vi "Create Queues.vi"(8 "error in (no error)":errorcluster) -> (0 "error out":errorcluster, 3 "Message Queues Out":T1)   [LabVIEW 2018]
uses:
  Pfizer Timed Seq/Software/support/Message Queue/Message Cluster.ctl
  Pfizer Timed Seq/Software/support/Message Queue/Enqueue Message (Single).vi
  Pfizer Timed Seq/Software/support/Message Queue/Message Queue.lvlib
panel:
  in  "Message Queues In":T1
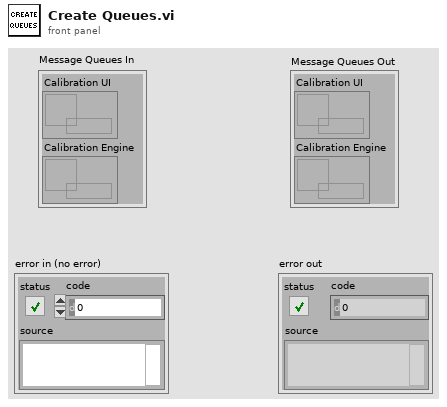
[diagram p1: front panel]
types:
  T1 = cluster{"Calibration UI":refnum<queue>, "Calibration Engine":refnum<queue>}
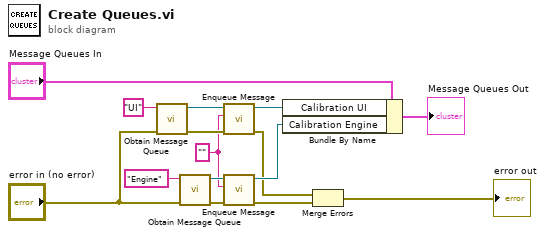
[diagram p0: block diagram]
diagram:
  w1 = "" ("Message")
  n1 = call "Obtain Message Queue.vi"("error in (no error)"="error in (no error)", "name (unnamed)"="UI") -> ("error out"=w12:errorcluster, "Message Queue"=w13:refnum<queue>)  [unwired: 8 in]
  n2 = call "Obtain Message Queue.vi"("error in (no error)"="error in (no error)", "name (unnamed)"="Engine") -> ("error out"=w14:errorcluster, "Message Queue"=w15:refnum<queue>)  [unwired: 8 in]
  n3 = call-poly "Enqueue Message.vi"("error in (no error)"=w12, "Message"=w1, "Message Queue"=w13) -> ("error out"=w4:errorcluster, "dup Message Queue"=w10:refnum<queue>)  [unwired: 7 in]
  n4 = call-poly "Enqueue Message.vi"("error in (no error)"=w14, "Message"=w1, "Message Queue"=w15) -> ("error out"=w3:errorcluster, "dup Message Queue"=w9:refnum<queue>)  [unwired: 7 in]
  n5 = Bundle By Name(cluster="Message Queues In", "Calibration UI"=w10, "Calibration Engine"=w9) -> (→"Message Queues Out":T1)
  n6 = Merge Errors(w4, w3) -> (→"error out":errorcluster)
